vi "Simple Video.vi"() -> ()   [LabVIEW 2014]
doc: "Very simple example showing how to use the base VIs to control the AR Drone and receive and display video data."
uses:
  Resources/Global.vi
panel:
  in  "milliseconds to wait":u32=25
  out "error out 3":errorcluster
  out "Video Stream 2":picture
  # "Do NOT un this VI. Instead run \"AR.Drone MAIN.vi\" and select the name of this VI in the dop-down menu at the Steup tab"
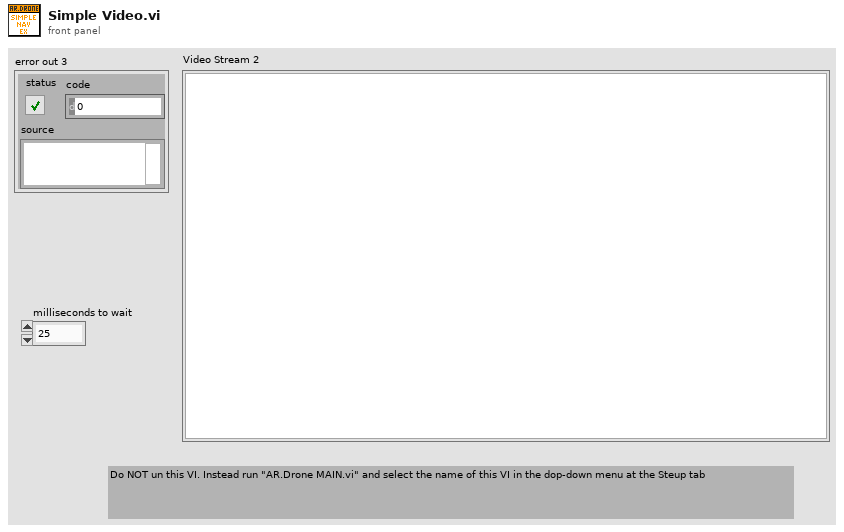
[diagram p1: front panel]
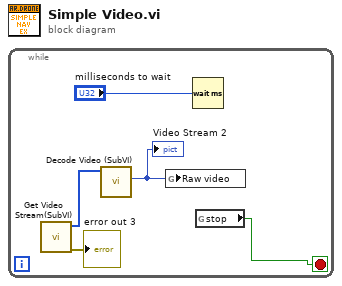
[diagram p0: block diagram]
diagram:
  n1 = while {
    stop <- w1 stop-if-true
    n2 = call "Get Video Stream(SubVI).vi"() -> ("error out"=→"error out 3":errorcluster, "ImgData"=w4:u8[])  [unwired: 10 in]
    n3 = call "Decode Video (SubVI).vi"("ImgData"=w4) -> ("new picture"=w3:picture)  [unwired: 9 in, 1 out]
    "Video Stream 2" <- w3
    n4 = global write "Global.vi" "Raw video"(w3) -> ()
    n5 = Wait (ms)(milliseconds to wait="milliseconds to wait") -> ()  [unwired: 1 out]
    n6 = global read "Global.vi" "stop"() -> (w1:bool)
  }
